vi "CreateCoordinateSystem.vi"(6 "error in (no error)":errorcluster, 8 "Coordinate System In":T1 {"Measurement System"."Axis Reference" items=["Direct", "Indirect"]; "Measurement System"."Angle (deg)" format="%.2f"; "Measurement System"."Origin"."Y" format="%.2f"; "Measurement System"."Origin"."X" format="%.2f"; "Reference System"."Axis Reference" items=["Direct", "Indirect"]; "Reference System"."Angle (deg)" format="%.2f"; "Reference System"."Origin"."Y" format="%.2f"; "Reference System"."Origin"."X" format="%.2f"}, 9 "Image":T2) -> (0 "error out":errorcluster, 1 "Y":sgl, 2 "ImageOut":T2(plugin-control), 3 "output cluster":T1 {"Measurement System"."Axis Reference" items=["Direct", "Indirect"]; "Measurement System"."Angle (deg)" format="%.2f"; "Measurement System"."Origin"."Y" format="%.2f"; "Measurement System"."Origin"."X" format="%.2f"; "Reference System"."Axis Reference" items=["Direct", "Indirect"]; "Reference System"."Angle (deg)" format="%.2f"; "Reference System"."Origin"."Y" format="%.2f"; "Reference System"."Origin"."X" format="%.2f"}, 4 "X":sgl)   [LabVIEW 2017]
uses:
  <vilib>/vision/Image Controls.llb/IMAQ Image.ctl
  <vilib>/vision/NI_Vision_Development_Module.lvlib
panel:
  out "Point1 (Real-World) 3":cluster{"X":sgl, "Y":sgl}
  out "Point1 (Real-World) 2":cluster{"X":sgl, "Y":sgl}
  out "Point2 (Real-World)":cluster{"X":sgl, "Y":sgl}
  out "Point1 (Real-World)":cluster{"X":sgl, "Y":sgl}
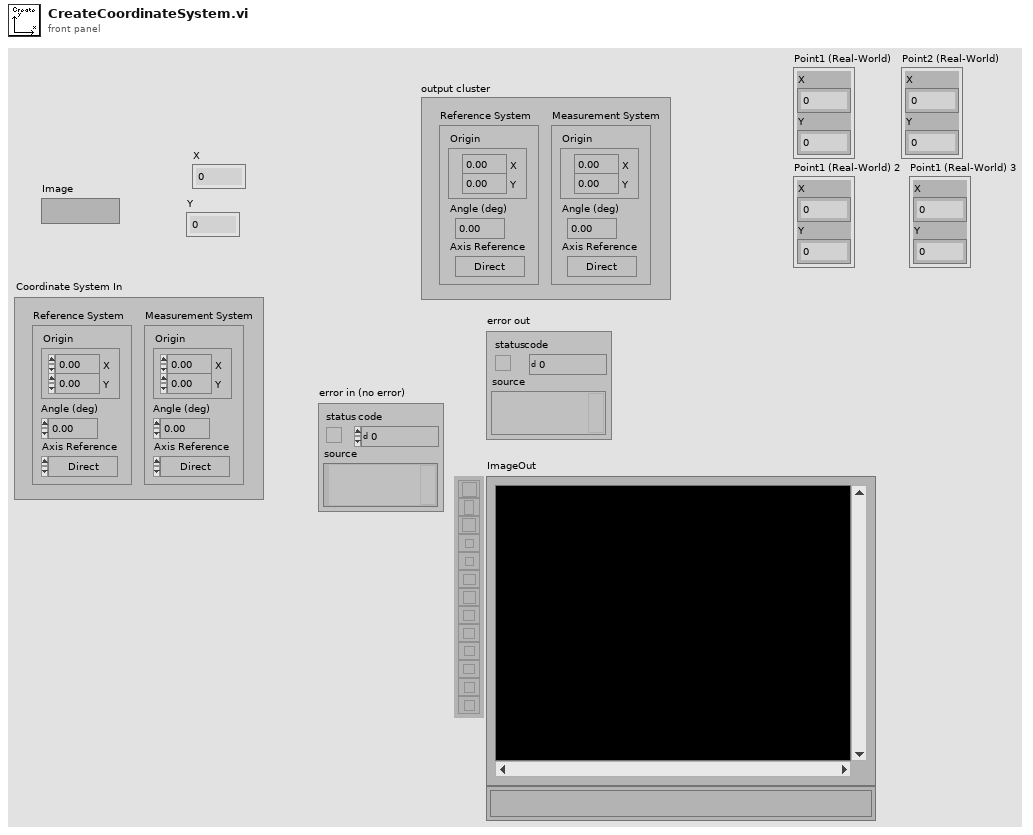
[diagram p1: front panel]
types:
  T1 = typedef "IMAQ Coordinate System" = cluster{"Reference System":cluster{"Origin":cluster{"X":sgl, "Y":sgl}, "Angle (deg)":sgl, "Axis Reference":u32}, "Measurement System":cluster{"Origin":cluster{"X":sgl, "Y":sgl}, "Angle (deg)":sgl, "Axis Reference":u32}}
  T2 = typedef "IMAQ Image.ctl" = refnum<image>
  T3 = cluster{"Point1 (Pixels)":cluster{"X":sgl, "Y":sgl}, "Point2 (Pixels)":cluster{"X":sgl, "Y":sgl}, "Point1 (Real-World)":cluster{"X":sgl, "Y":sgl}, "Point2 (Real-World)":cluster{"X":sgl, "Y":sgl}, "Angle (Pixel)":dbl, "Angle (Real-World)":dbl, "Score":dbl, "Straightness":dbl, "Average SNR (db)":dbl, "Calibration Valid":bool}[]
  T4 = cluster{"Straight Edges[0]":cluster{"Point1 (Pixels)":cluster{"X":sgl, "Y":sgl}, "Point2 (Pixels)":cluster{"X":sgl, "Y":sgl}, "Point1 (Real-World)":cluster{"X":sgl, "Y":sgl}, "Point2 (Real-World)":cluster{"X":sgl, "Y":sgl}, "Angle (Pixel)":dbl, "Angle (Real-World)":dbl, "Score":dbl, "Straightness":dbl, "Average SNR (db)":dbl, "Calibration Valid":bool}, "Straight Edges[1]":cluster{"Point1 (Pixels)":cluster{"X":sgl, "Y":sgl}, "Point2 (Pixels)":cluster{"X":sgl, "Y":sgl}, "Point1 (Real-World)":cluster{"X":sgl, "Y":sgl}, "Point2 (Real-World)":cluster{"X":sgl, "Y":sgl}, "Angle (Pixel)":dbl, "Angle (Real-World)":dbl, "Score":dbl, "Straightness":dbl, "Average SNR (db)":dbl, "Calibration Valid":bool}, "Straight Edges[2]":cluster{"Point1 (Pixels)":cluster{"X":sgl, "Y":sgl}, "Point2 (Pixels)":cluster{"X":sgl, "Y":sgl}, "Point1 (Real-World)":cluster{"X":sgl, "Y":sgl}, "Point2 (Real-World)":cluster{"X":sgl, "Y":sgl}, "Angle (Pixel)":dbl, "Angle (Real-World)":dbl, "Score":dbl, "Straightness":dbl, "Average SNR (db)":dbl, "Calibration Valid":bool}, "Straight Edges[3]":cluster{"Point1 (Pixels)":cluster{"X":sgl, "Y":sgl}, "Point2 (Pixels)":cluster{"X":sgl, "Y":sgl}, "Point1 (Real-World)":cluster{"X":sgl, "Y":sgl}, "Point2 (Real-World)":cluster{"X":sgl, "Y":sgl}, "Angle (Pixel)":dbl, "Angle (Real-World)":dbl, "Score":dbl, "Straightness":dbl, "Average SNR (db)":dbl, "Calibration Valid":bool}, "Straight Edges[4]":cluster{"Point1 (Pixels)":cluster{"X":sgl, "Y":sgl}, "Point2 (Pixels)":cluster{"X":sgl, "Y":sgl}, "Point1 (Real-World)":cluster{"X":sgl, "Y":sgl}, "Point2 (Real-World)":cluster{"X":sgl, "Y":sgl}, "Angle (Pixel)":dbl, "Angle (Real-World)":dbl, "Score":dbl, "Straightness":dbl, "Average SNR (db)":dbl, "Calibration Valid":bool}, "Straight Edges[5]":cluster{"Point1 (Pixels)":cluster{"X":sgl, "Y":sgl}, "Point2 (Pixels)":cluster{"X":sgl, "Y":sgl}, "Point1 (Real-World)":cluster{"X":sgl, "Y":sgl}, "Point2 (Real-World)":cluster{"X":sgl, "Y":sgl}, "Angle (Pixel)":dbl, "Angle (Real-World)":dbl, "Score":dbl, "Straightness":dbl, "Average SNR (db)":dbl, "Calibration Valid":bool}, "Straight Edges[6]":cluster{"Point1 (Pixels)":cluster{"X":sgl, "Y":sgl}, "Point2 (Pixels)":cluster{"X":sgl, "Y":sgl}, "Point1 (Real-World)":cluster{"X":sgl, "Y":sgl}, "Point2 (Real-World)":cluster{"X":sgl, "Y":sgl}, "Angle (Pixel)":dbl, "Angle (Real-World)":dbl, "Score":dbl, "Straightness":dbl, "Average SNR (db)":dbl, "Calibration Valid":bool}, "Straight Edges[7]":cluster{"Point1 (Pixels)":cluster{"X":sgl, "Y":sgl}, "Point2 (Pixels)":cluster{"X":sgl, "Y":sgl}, "Point1 (Real-World)":cluster{"X":sgl, "Y":sgl}, "Point2 (Real-World)":cluster{"X":sgl, "Y":sgl}, "Angle (Pixel)":dbl, "Angle (Real-World)":dbl, "Score":dbl, "Straightness":dbl, "Average SNR (db)":dbl, "Calibration Valid":bool}, "Straight Edges[8]":cluster{"Point1 (Pixels)":cluster{"X":sgl, "Y":sgl}, "Point2 (Pixels)":cluster{"X":sgl, "Y":sgl}, "Point1 (Real-World)":cluster{"X":sgl, "Y":sgl}, "Point2 (Real-World)":cluster{"X":sgl, "Y":sgl}, "Angle (Pixel)":dbl, "Angle (Real-World)":dbl, "Score":dbl, "Straightness":dbl, "Average SNR (db)":dbl, "Calibration Valid":bool}}
  T5 = cluster{"Point1 (Pixels)":cluster{"X":sgl, "Y":sgl}, "Point2 (Pixels)":cluster{"X":sgl, "Y":sgl}, "Point1 (Real-World)":cluster{"X":sgl, "Y":sgl}, "Point2 (Real-World)":cluster{"X":sgl, "Y":sgl}, "Angle (Pixel)":dbl, "Angle (Real-World)":dbl, "Score":dbl, "Straightness":dbl, "Average SNR (db)":dbl, "Calibration Valid":bool}
  T6 = cluster{"Point1 (Real-World)":cluster{"X":sgl, "Y":sgl}, "Point2 (Real-World)":cluster{"X":sgl, "Y":sgl}}
  T7 = cluster{"Origin":cluster{"X":sgl, "Y":sgl}, "Angle (deg)":sgl, "Axis Reference":u32}
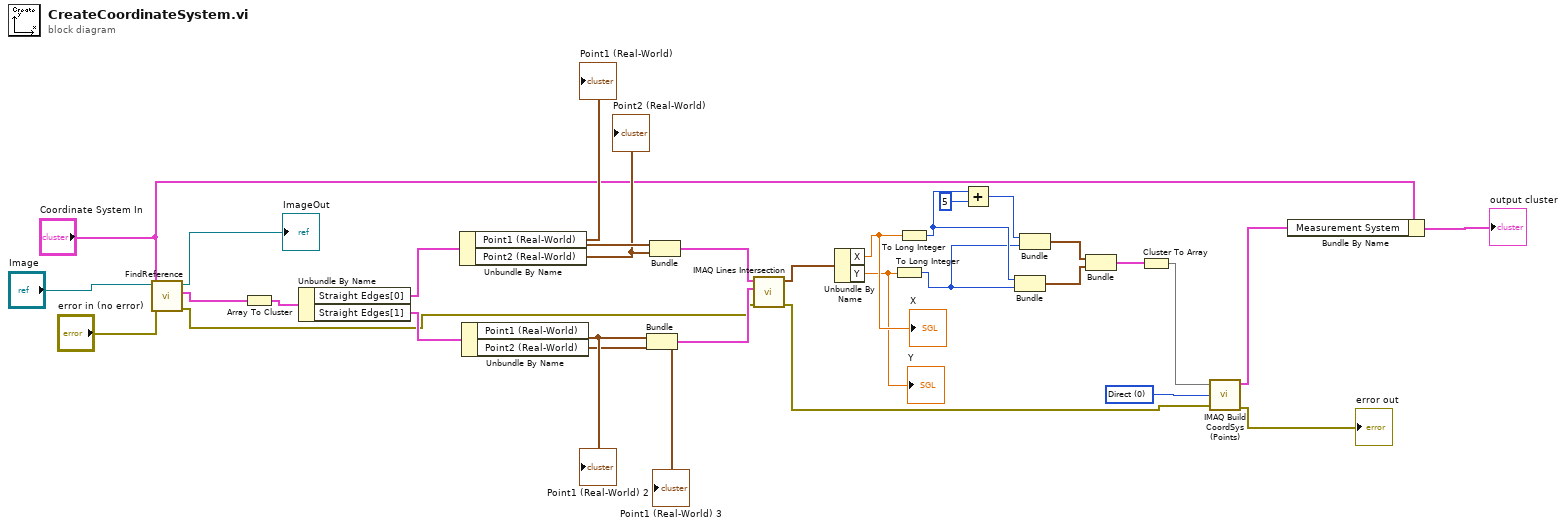
[diagram p0: block diagram]
diagram:
  w12 = u32 0 items=["Direct", "Indirect"] ("Axis Reference")
  n1 = call "FindReference.vi"("error in (no error)"="error in (no error)", "Coordinate System"="Coordinate System In", "Image"="Image") -> ("error out"=w9:errorcluster, "Straight Edges"=w31:T3, "Image 2"=→"ImageOut":T2)  [unwired: 6 in]
  n2 = Array To Cluster(array=w31) -> (cluster=w30:T4)
  n3 = Unbundle By Name(w30) -> ("Straight Edges[0]"=w29:T5, "Straight Edges[1]"=w28:T5)
  n4 = Unbundle By Name(w29) -> ("Point1 (Real-World)"=w27:cluster{"X":sgl, "Y":sgl}, "Point2 (Real-World)"=w26:cluster{"X":sgl, "Y":sgl})
  "Point1 (Real-World)" <- w27
  "Point2 (Real-World)" <- w26
  n5 = Unbundle By Name(w28) -> ("Point1 (Real-World)"=w25:cluster{"X":sgl, "Y":sgl}, "Point2 (Real-World)"=w24:cluster{"X":sgl, "Y":sgl})
  "Point1 (Real-World) 2" <- w25
  "Point1 (Real-World) 3" <- w24
  n6 = Bundle("Point1 (Real-World)"=w25, "Point2 (Real-World)"=w24) -> (w22:T6)  [unwired: 1 in]
  n7 = Bundle("Point1 (Real-World)"=w27, "Point2 (Real-World)"=w26) -> (w23:T6)  [unwired: 1 in]
  n8 = call "IMAQ Lines Intersection"("error in (no error)"=w9, "Line 2"=w22, "Line 1"=w23) -> ("error out"=w8:errorcluster, "Intersection Point"=w21:cluster{"X":sgl, "Y":sgl})  [unwired: 6 in, 1 out]
  n9 = Unbundle By Name(w21) -> ("X"=w2:sgl, "Y"=w1:sgl)
  "X" <- w2
  "Y" <- w1
  n10 = To Long Integer(number=w1) -> (32bit integer=w17:i32)
  n11 = To Long Integer(number=w2) -> (32bit integer=w19:i32)
  n12 = Add(x=w19, y=5) -> (x+y=w18:i32)
  n13 = Bundle(w19, w17) -> (w15:cluster{i32, i32})  [unwired: 1 in]
  n14 = Bundle(w18, w17) -> (w16:cluster{i32, i32})  [unwired: 1 in]
  n15 = Bundle(w16, w15) -> (w14:cluster{cluster{i32, i32}, cluster{i32, i32}})  [unwired: 1 in]
  n16 = Cluster To Array(cluster=w14) -> (array=w13:cluster{i32, i32}[])
  n17 = call "IMAQ Build CoordSys (Points)"("Reference Points"=w13, "Axis Reference"=w12, "error in (no error)"=w8) -> ("Coordinate System"=w4:T7, "error out"=→"error out":errorcluster)  [unwired: 2 in]
  n18 = Bundle By Name(cluster="Coordinate System In", "Measurement System"=w4) -> (→"output cluster":T1)
